vi "Emballage_NumSerieParSemaine.vi"(8 "Error in":errorcluster caption="Error in (no error)", 9 "fichier erroné":bool, 10 "texte":string="hello", 11 "ID_ARTICLE":string) -> (0 "Error out":errorcluster)   [LabVIEW 2020]
uses:
  Modules/FS/60_FS_Controles/60_FS_SetGet.ctl
  <vilib>/Utility/NIReport.llb/Report Type.ctl
  <vilib>/addons/_office/_exclsub.llb/font.ctl
  <vilib>/Utility/NIReport.llb/Append Report Text (str wrap).vi
  <vilib>/Utility/NIReport.llb/NI_report.lvclass
  <vilib>/drjdpowell/SQLite Library/SQL Connection/Connection.lvclass
  <vilib>/Utility/NIReport.llb/NI_ReportGenerationCore.lvlib
  <vilib>/Utility/NIReport.llb/Word/NI_Word.lvclass
  <vilib>/addons/_office/NI_ReportGenerationToolkit.lvlib
  <vilib>/drjdpowell/SQLite Library/SQL Connection/Open (path).vi
panel:
  out "Result Set":string[][](table) caption="Result Set (from first statement with results)"
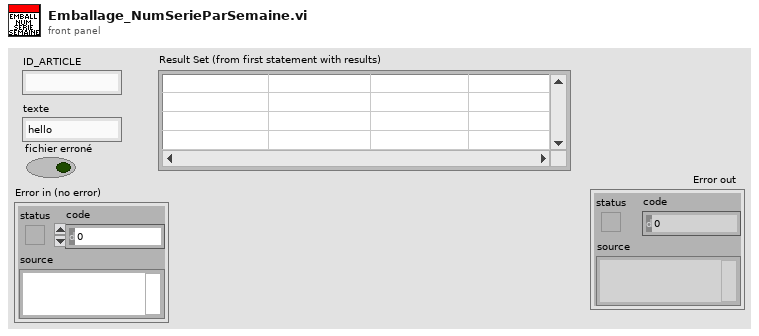
[diagram p1: front panel]
types:
  T1 = typedef "60_FS_SetGet.ctl" = enum16{"set", "get"}
  T2 = enum16{"open", "replace", "create", "open or create", "replace or create", "replace or create with confirmation"}
  T3 = enum16{"maximized", "minimized", "normal", "no change"}
  T4 = cluster{"alignment":enum16{"Left", "Centered", "Right", "Justify"}, "left":dbl, "right":dbl, "special":enum16{"(none)", "First line", "Hanging"}, "by":dbl, "before":dbl, "after":dbl, "line spacing":enum16{"Single", "1,5 lines", "Double", "At least", "Exactly", "Multiple"}, "at":dbl}
  T5 = typedef "NI_ReportGenerationToolkit.lvlib/font.ctl" = cluster{"font name":string, "font size":dbl, "bold":u16, "italic":u16, "underline":u16, "strike through":u16, "font color":u32}
  T6 = typedef "NI_ReportGenerationCore.lvlib/Report Type.ctl" = enum16{"HTML", "Word", "Excel"}
  T7 = typedef "60_FS_CLT_Chemins.ctl" = cluster{"Racine_local":path, "Racine_reseau":path, "Racine_Support_Application":path, "Fichier_Journalisation":path, "Connexion_BDD_VSX":path, "Connexion_BDD_PLZ":path}
  T8 = cluster{"Admin-réseau":path, "XML-Réseau":path, " Résultat tests-Réseau":path, " Archive prôbleme-Réseau":path, " Archive Test  Local":path}
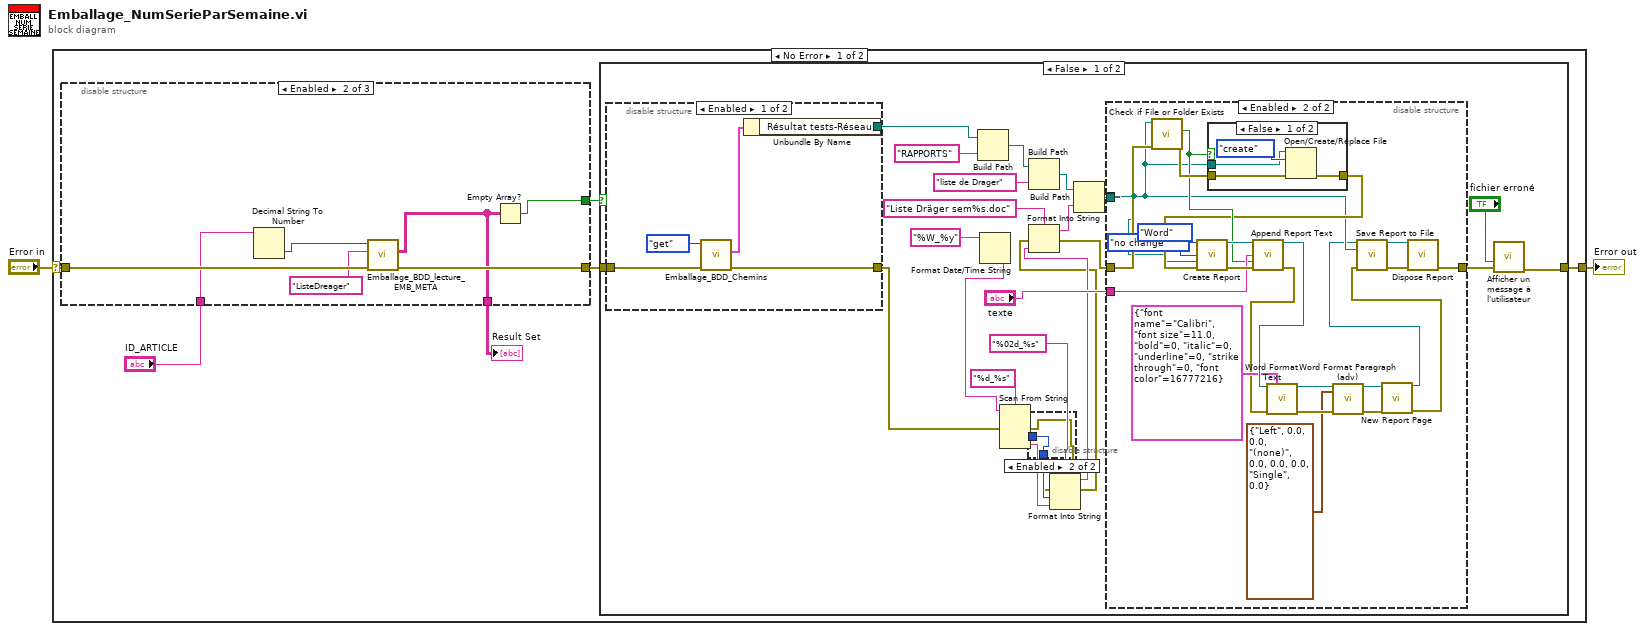
[diagram p0: block diagram]
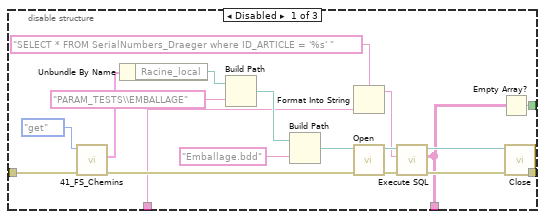
[diagram p2: hidden frame]
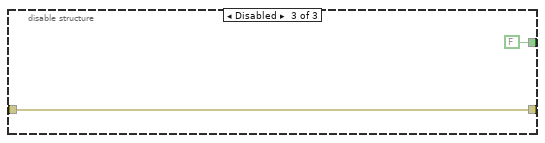
[diagram p3: hidden frame]
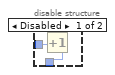
[diagram p4: hidden frame]
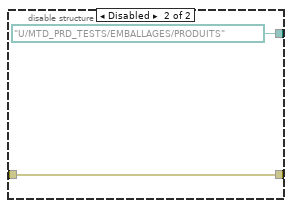
[diagram p5: hidden frame]
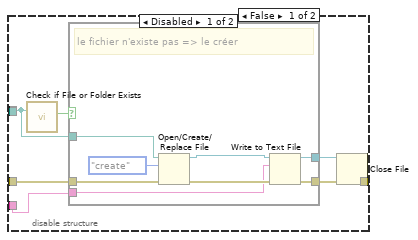
[diagram p6: hidden frame]
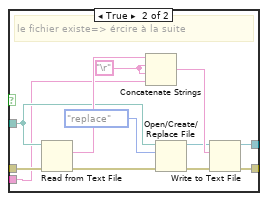
[diagram p7: hidden frame]
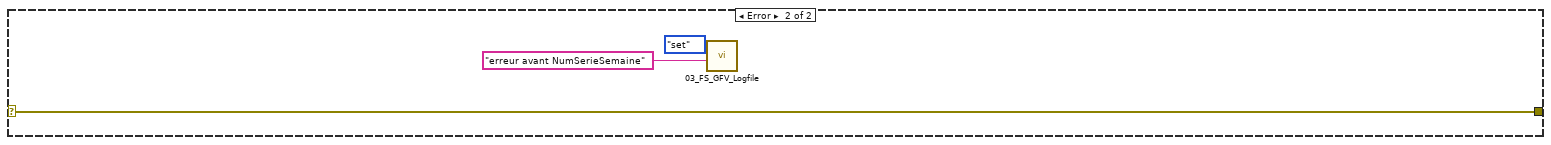
[diagram p10: hidden frame]
diagram:
  n1 = case shown="No Error" "Error in" {
    selector: "Error in" -> [w6 w130]
    tunnel: [w5 w130] -> w1
    frame No Error {
      n2 = disable-structure shown="Enabled" {
        disable-tunnel: [w13 w30 FALSE ("empty?")] -> w8
        disable-tunnel: [w12 w33 w35] -> w7
        disable-tunnel: w6 -> [w11 w34 w35]
        disable-tunnel: "ID_ARTICLE" -> [w10 w32 _]
        disable-tunnel: [w9 w29 _] -> w3
        frame Disabled {
          n3 = call "41_FS_Chemins.vi"("error in (no error)"=w11, "SetGet"=60_FS_SetGet."get") -> ("error out"=w25:errorcluster, "CLT_Chemins_out"=w17:T7)  [unwired: 8 in]
          n4 = Unbundle By Name(w17) -> ("Racine_local"=w19:path)
          n5 = Build Path(base path=w19, name or relative path="PARAM_TESTS\\EMBALLAGE" ("nom ou chemin relatif")) -> (appended path=w21:path)
          n6 = Build Path(base path=w21, name or relative path="Emballage.bdd" ("nom ou chemin relatif")) -> (appended path=w27:path)
          n7 = Format Into String(format string="SELECT * FROM SerialNumbers_Draeger where ID_ARTICLE = '%s' " ("SQL"), w10) -> (resulting string=w22:string)  [unwired: 2 in, 1 out]
          n8 = call-poly <vilib>:"Open.vi"("error in (no error)"=w25, "db file"=w27) -> ("error out"=w24:errorcluster, "SQLite Connection"=w26:refnum<class "Connection.lvclass">)  [unwired: 8 in]
          n9 = call <vilib>:"Execute SQL.vi"("error in (no error)"=w24, "SQL"=w22, "SQLite Connection in"=w26) -> ("error out"=w14:errorcluster, "Result Set"=w9:string[][], "SQLite Connection"=w15:refnum<class "Connection.lvclass">)  [unwired: 5 in, 1 out]
          n10 = Empty Array?(array=w9) -> (empty?=w13:bool)
          n11 = call-dynamic "Close.vi"("error in (no error)"=w14, "SQLite Connection in"=w15) -> ("error out"=w12:errorcluster)  [unwired: 9 in]
        }
        frame Enabled {
          n12 = Decimal String To Number(string=w32) -> (number=w28:i32)  [unwired: 2 in, 1 out]
          n13 = call "Emballage_BDD_lecture_EMB_META.vi"("Error in"=w34, "CLE"="ListeDreager", "ID_ARTICLE_GPAO"=w28) -> ("Error out"=w33:errorcluster, "Result Set"=w29:string[][])  [unwired: 6 in, 1 out]
          n14 = Empty Array?(array=w29) -> (empty?=w30:bool)
        }
        frame Disabled {
        }
      }
      "Result Set" <- w3
      n15 = case shown="False" w8 {
        tunnel: w7 -> [w53 w127]
        tunnel: [w49 w127] -> w5
        frame False {
          n16 = disable-structure shown="Enabled" {
            disable-tunnel: [w69 path "U:/MTD_PRD_TESTS/EMBALLAGES/PRODUITS" ("Résultat tests-Réseau")] -> w60
            disable-tunnel: w53 -> [w66 w70]
            disable-tunnel: [w65 w70] -> w40
            frame Enabled {
              n17 = call "Emballage_BDD_Chemins.vi"("error in (no error)"=w66, "SetGet"=60_FS_SetGet."get") -> ("error out"=w65:errorcluster, "CLT_Chemins_out"=w68:T8)  [unwired: 8 in]
              n18 = Unbundle By Name(w68) -> ("Résultat tests-Réseau"=w69:path)
            }
            frame Disabled {
            }
          }
          n19 = Build Path(base path=w60, name or relative path="RAPPORTS" ("nom ou chemin relatif")) -> (appended path=w59:path)
          n20 = Format Date/Time String(time format string (%c)="%W_%y" ("chaîne de format de l'heure (%c)")) -> (date/time string=w42:string)  [unwired: 2 in]
          n21 = Scan From String(format string="%d_%s" ("chaîne de format"), input string=w42, error in=w40) -> (error out=w39:errorcluster, output 1=w47:i32, output 2=w44:string)  [unwired: 3 in, 2 out]
          n22 = Build Path(base path=w59, name or relative path="liste de Drager" ("nom ou chemin relatif")) -> (appended path=w55:path)
          n23 = disable-structure shown="Enabled" {
            disable-tunnel: w47 -> [w63 w64]
            disable-tunnel: [w62 w64] -> w45
            frame Disabled {
              n24 = Increment(x=w63) -> (x+1=w62:i32)
            }
            frame Enabled {
            }
          }
          n25 = Format Into String(format string="%02d_%s" ("chaîne de format"), error in=w39, w45, w44) -> (resulting string=w41:string, error out=w38:errorcluster)  [unwired: 1 in]
          n26 = Format Into String(format string="Liste Dräger sem%s.doc", error in=w38, w41) -> (resulting string=w54:string, error out=w37:errorcluster)  [unwired: 1 in]
          n27 = Build Path(base path=w55, name or relative path=w54) -> (appended path=w51:path)
          n28 = disable-structure shown="Enabled" {
            disable-tunnel: w51 -> [w77 w110]
            disable-tunnel: [w74 w118] -> w50
            disable-tunnel: w37 -> [w73 w114]
            disable-tunnel: "texte" -> [w72 w115]
            disable-tunnel: w51 -> [_ _]
            frame Disabled {
              n29 = call <vilib>:"Check if File or Folder Exists.vi"("path"=w77) -> ("file or folder exists?"=w78:bool)  [unwired: 8 in, 2 out]
              n30 = case shown="False" w78 {
                tunnel: w77 -> [w86 w93]
                tunnel: [w83 w97] -> w76
                tunnel: [w82 w96] -> w75
                tunnel: w73 -> [w80 w91]
                tunnel: w72 -> [w79 w87]
                frame False {
                  # "le fichier n'existe pas => le créer"
                  n31 = Open/Create/Replace File(file path (use dialog)=w86, error in=w80, operation (0:open)=T2."create" ("opération (0 : open)")) -> (refnum out=w84:refnum<file>, error out=w81:errorcluster)  [unwired: 3 in, 1 out]
                  n32 = Write to Text File(file (use dialog)=w84, text=w79, error in=w81) -> (refnum out=w82:refnum<file>, error out=w83:errorcluster)  [unwired: 1 in, 1 out]
                }
                frame True {
                  w88 = "\r"
                  # "le fichier existe=> ércire à la suite"
                  n33 = Read from Text File(file (use dialog)=w93, error in=w91) -> (text=w95:string, error out=w90:errorcluster)  [unwired: 2 in, 2 out]
                  n34 = Concatenate Strings(w95, w88, w88, w87) -> (w94:string)
                  n35 = Open/Create/Replace File(file path (use dialog)=w93, error in=w90, operation (0:open)=T2."replace" ("opération (0 : open)")) -> (refnum out=w92:refnum<file>, error out=w89:errorcluster)  [unwired: 3 in, 1 out]
                  n36 = Write to Text File(file (use dialog)=w92, text=w94, error in=w89) -> (refnum out=w96:refnum<file>, error out=w97:errorcluster)  [unwired: 1 in, 1 out]
                }
              }
              n37 = Close File(refnum=w75, error in=w76) -> (error out=w74:errorcluster)  [unwired: 1 out]
            }
            frame Enabled {
              n38 = call <vilib>:"Check if File or Folder Exists.vi"("error in (no error)"=w114, "path"=w110) -> ("error out"=w113:errorcluster, "file or folder exists?"=w112:bool)  [unwired: 7 in, 1 out]
              n39 = case shown="False" w112 {
                tunnel: w110 -> [w124 _]
                tunnel: w113 -> [w123 w126]
                tunnel: [w122 w126] -> w111
                frame False {
                  n40 = Open/Create/Replace File(file path (use dialog)=w124, error in=w123, operation (0:open)=T2."create" ("opération (0 : open)")) -> (error out=w122:errorcluster)  [unwired: 3 in, 2 out]
                }
                frame True {
                }
              }
              n41 = call <vilib>:"Create Report.vi"("window state (normal)"=T3."no change", "report type"=Report_Type."Word", "template (empty)"=w110, "error in (no error)"=w111) -> ("report out"=w116:refnum<class "NI_report.lvclass">, "error out"=w120:errorcluster)  [unwired: 10 in]
              n42 = call-poly <vilib>:"Append Report Text.vi"("report in"=w116, "text"=w115, "append on new line? (F)"=w112, "error in (no error)"=w120) -> ("report out"=w109:refnum<class "NI_report.lvclass">, "error out"=w107:errorcluster)  [unwired: 8 in, 2 out]
              n43 = call <vilib>:"Word Format Text.vi"("report in"=w109, "font"=T5 {"font name"="Calibri", "font size"=11.0, "bold"=0, "italic"=0, "underline"=0, "strike through"=0, "font color"=16777216}, "error in (no error)"=w107) -> ("report out"=w105:refnum<class "NI_report.lvclass">, "error out"=w106:errorcluster)  [unwired: 11 in]
              n44 = call <vilib>:"Word Format Paragraph (adv).vi"("report in"=w105, "indent and spacing"=T4 {"alignment"=enum."Left", "left"=0.0, "right"=0.0, "special"=enum."(none)", "by"=0.0, "before"=0.0, "after"=0.0, "line spacing"=enum."Single", "at"=0.0}, "error in (no error)"=w106) -> ("report out"=w102:refnum<class "NI_report.lvclass">, "error out"=w103:errorcluster)  [unwired: 11 in]
              n45 = call-dynamic "New Report Page.vi"("report in"=w102, "error in (no error)"=w103) -> ("report out"=w101:refnum<class "NI_report.lvclass">, "error out"=w100:errorcluster)  [unwired: 12 in]
              n46 = call-dynamic "Save Report to File.vi"("report in"=w101, "report file path"=w110, "error in (no error)"=w100) -> ("report out"=w117:refnum<class "NI_report.lvclass">, "error out"=w119:errorcluster)  [unwired: 11 in]
              n47 = call-dynamic "Dispose Report.vi"("report in"=w117, "error in (no error)"=w119) -> ("error out"=w118:errorcluster)  [unwired: 13 in]
            }
          }
          n48 = call "Afficher un message à l'utilisateur"("error in (no error)"=w50, "Enable"="fichier erroné") -> ("error out"=w49:errorcluster)  [unwired: 8 in, 1 out]
        }
        frame True {
          # "Tableau vide donc pas fichier liste par semaine"
        }
      }
    }
    frame Error {
      n49 = call "03_FS_GFV_Logfile.vi"("Chaîne"="erreur avant NumSerieSemaine", "States"=60_FS_SetGet."set") -> ()  [unwired: 8 in, 2 out]
    }
  }
  "Error out" <- w1
